vi "Update Properties in SysDef debug.vi"(8 "error in (no error)":errorcluster, 10 "Changed Properties":T1[](array[typedef]), 11 "Node Ptr":T2 format="%.0x") -> (0 "error out":errorcluster, 3 "Item Ref out":T2 format="%.0x")   [LabVIEW 2019]
doc: "Check which property value was changed and update that."
uses:
  SLSC EDS API/JSON parsing/propertySysDefPage.ctl
  <vilib>/NI VeriStand/Custom Device API/Custom Device Item Ref.ctl
  Shared/Constants.vi
  SLSC EDS API/JSON parsing/property.ctl
  <vilib>/NI VeriStand/Custom Device API/Custom Device API.lvlib
  Shared/SLSC EDS Shared.lvlib
  <vilib>/NI VeriStand/Custom Device API/Get Item Property (Variant).vi
panel:
  out "Array":bool[](array[boolean])
  in  "Properties":T1[](array[typedef])
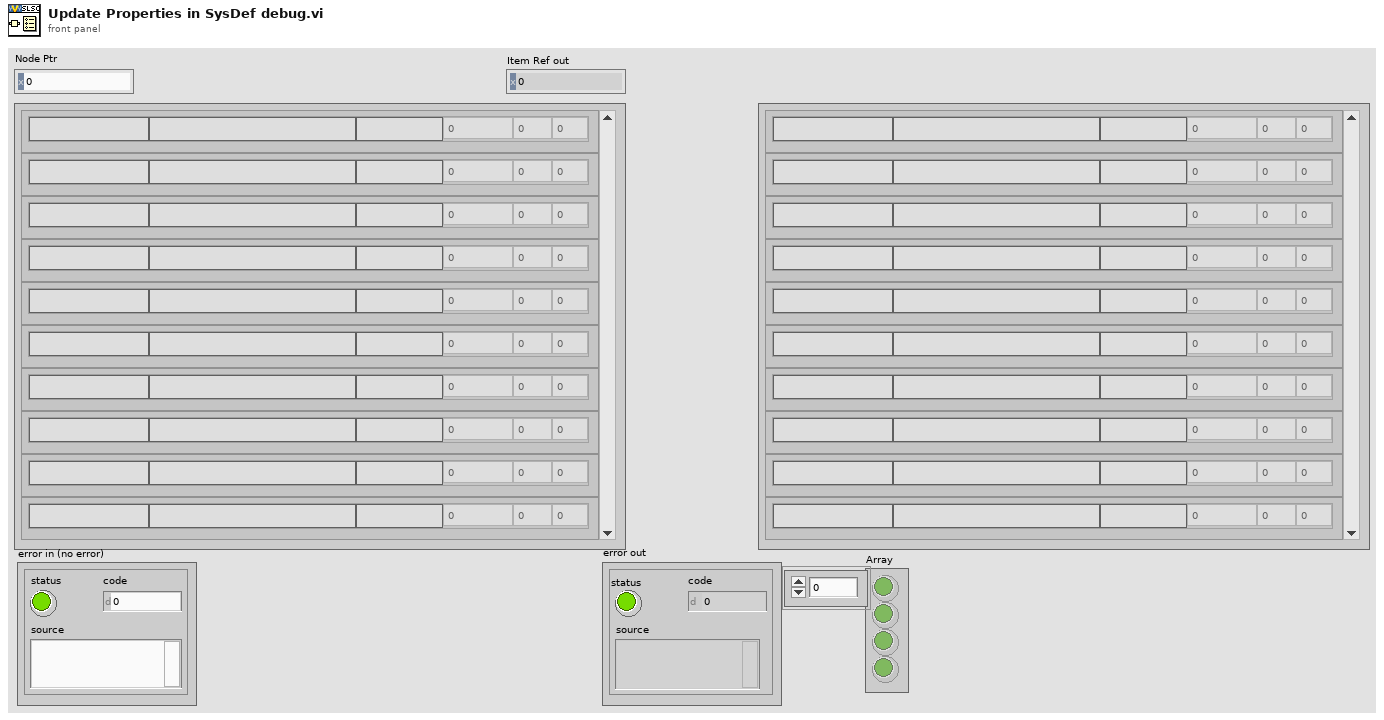
[diagram p1: front panel]
types:
  T1 = typedef "propertySysDefPage.ctl" = cluster{"name":string, "description-en":string, "dataType":string, "value":dbl, "min":dbl, "max":dbl}
  T2 = typedef "Custom Device API.lvlib/Custom Device Item Ref.ctl" = u64
  T3 = typedef "property.ctl" = cluster{"name":string, "description-en":string, "documentation-en":string, "dataType":string, "bitfield":string, "access":string, "scale":string, "value":variant, "min":variant, "max":variant, "default value":variant}
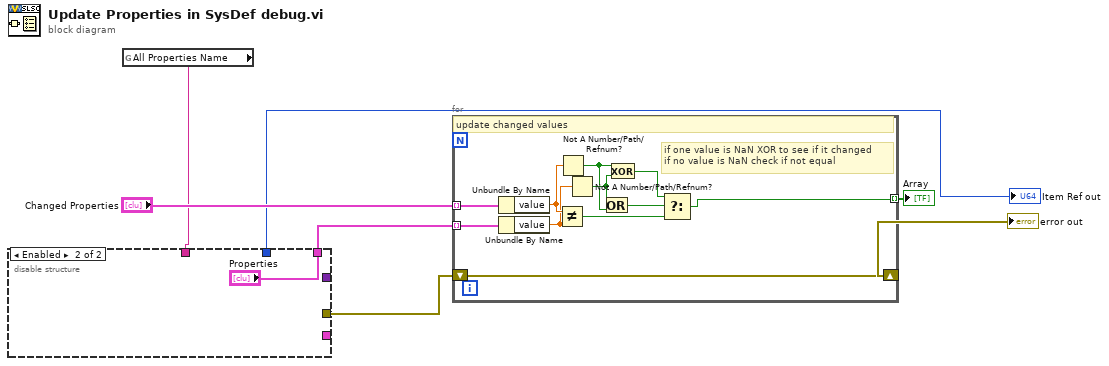
[diagram p0: block diagram]
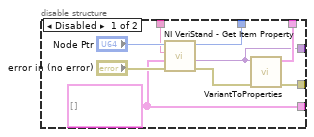
[diagram p2: hidden frame]
diagram:
  n1 = global read "Constants.vi" "All Properties Name"() -> (w4:string)
  n2 = disable-structure shown="Enabled" {
    disable-tunnel: [w13 "Properties"] -> w6
    disable-tunnel: [w12 _] -> w2
    disable-tunnel: [w11 _] -> _
    disable-tunnel: [w10 _] -> _
    disable-tunnel: [w9 _] -> w5
    disable-tunnel: w4 -> [w8 _]
    frame Disabled {
      w10 = T3[] [] ("properties")
      n3 = call-poly <vilib>:"NI VeriStand - Get Item Property.vi"("error in (no error)"="error in (no error)", "Default Value"=w10, "Property Name"=w8, "Item Ref in"="Node Ptr") -> ("error out"=w14:errorcluster, "Value"=w11:variant, "Item Ref out"=w9:T2)  [unwired: 4 in, 1 out]
      n4 = call "VariantToProperties.vi"("error in (no error)"=w14, "Variant"=w11) -> ("error out"=w12:errorcluster, "Properties"=w13:T1[])  [unwired: 8 in]
    }
    frame Enabled {
    }
  }
  "Item Ref out" <- w5
  n5 = for {
    tunnel: "Changed Properties" -> [w28] mode=indexing
    tunnel: w6 -> [w27] mode=indexing
    shift-right: [w26] -> w3
    shift-left: w2 -> [w26]
    tunnel: [w18] -> w1 mode=indexing
    # "if one value is NaN XOR to see if it changed\nif no value is NaN check if not equal"
    # "update changed values"
    n6 = Unbundle By Name(w28) -> ("value"=w25:dbl)
    n7 = Unbundle By Name(w27) -> ("value"=w24:dbl)
    n8 = Not Equal?(x=w25, y=w24) -> (x != y?=w19:bool)
    n9 = Not A Number/Path/Refnum?(number/path/refnum=w25) -> (NaN/Path/Refnum?=w22:bool)
    n10 = Not A Number/Path/Refnum?(number/path/refnum=w24) -> (NaN/Path/Refnum?=w23:bool)
    n11 = Or(x=w23, y=w22) -> (x .or. y?=w21:bool)
    n12 = Exclusive Or(1:w23, 2:w22) -> (0:w20:bool)
    n13 = Select(t=w20, s=w21, f=w19) -> (s? t:f=w18:bool)
  }
  "error out" <- w3
  "Array" <- w1
